vi "Helper_Timestamp (SubVI).vi"(11 "Labview Timestamp":timestamp=timestamp(2082862800 s since 1904-01-01) format="%<%H:%M:%S%3u\n%x>T") -> (1 "Unix Timestamp":dbl format="%#_16g", 2 "ThingworxTimestamp":dbl format="%#_16g", 3 "Thingworx Timestamp String":string)   [LabVIEW 2018]
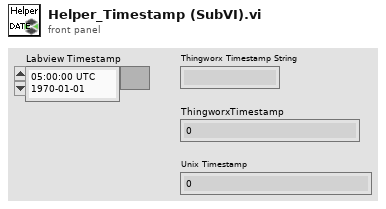
[diagram p1: front panel]
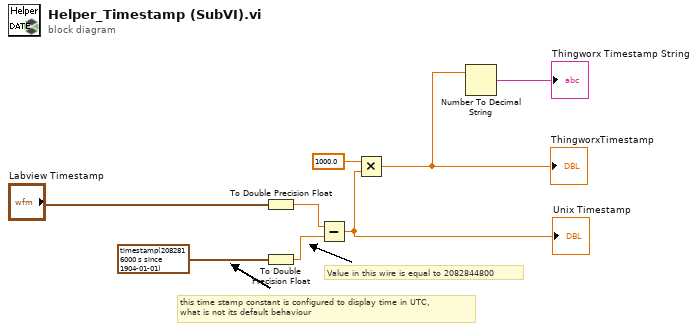
[diagram p0: block diagram]
diagram:
  # "Value in this wire is equal to 2082844800"
  # "this time stamp constant is configured to display time in UTC, \nwhat is not its default behaviour"
  n1 = To Double Precision Float(number="Labview Timestamp") -> (double precision float=w1:dbl)
  n2 = To Double Precision Float(number=timestamp(2082816000 s since 1904-01-01)) -> (double precision float=w2:dbl)
  n3 = Subtract(x=w1, y=w2) -> (x-y=w4:dbl)
  "Unix Timestamp" <- w4
  n4 = Multiply(x=1000.0, y=w4) -> (x*y=w7:dbl)
  "ThingworxTimestamp" <- w7
  n5 = Number To Decimal String(number=w7) -> (decimal integer string=→"Thingworx Timestamp String":string)  [unwired: 1 in]
